vi "4145 validate GUI.vi"(7 "advanced?":bool, 10 "error in (no error)":errorcluster, 11 "AdvancedConfig":T1={"X Axis Name"="", "X axis"=TRUE, "X scale"=TRUE, "Is X axis VAR 1?"=FALSE, "X Axis min"=0.0, "X Axis max"=1.0, "Y1 Axis Name"="", "Y1 scale"=TRUE, "Is VAR 2 used?"=FALSE, "# of steps for VAR 2"=0, "Y1 Axis min"=0.0, "Y1 Axis max"=0.01, "Y2 Axis Name"="", "Y2 axis"=FALSE, "Y2 scale"=TRUE, "Y2 Axis min"=0.0, "Y2 Axis max"=0.01} caption="Simple" {"Y2 Axis max" format="%^.3e"; "Y2 Axis min" format="%^.3e"; "Y1 Axis max" format="%^.3e"; "Y1 Axis min" format="%^.3e"; "X Axis max" format="%^.3e"; "X Axis min" format="%^.3e"}) -> (2 "error out":errorcluster, 3 "valid":bool)   [LabVIEW 2014]
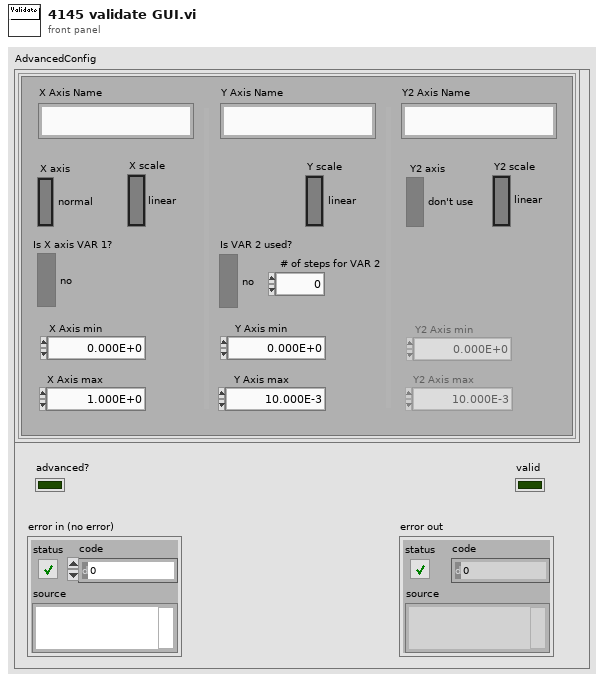
[diagram p1: front panel]
types:
  T1 = cluster{"X Axis Name":string, "X axis":bool, "X scale":bool, "Is X axis VAR 1?":bool, "X Axis min":dbl, "X Axis max":dbl, "Y1 Axis Name":string, "Y1 scale":bool, "Is VAR 2 used?":bool, "# of steps for VAR 2":u16, "Y1 Axis min":dbl, "Y1 Axis max":dbl, "Y2 Axis Name":string, "Y2 axis":bool, "Y2 scale":bool, "Y2 Axis min":dbl, "Y2 Axis max":dbl}
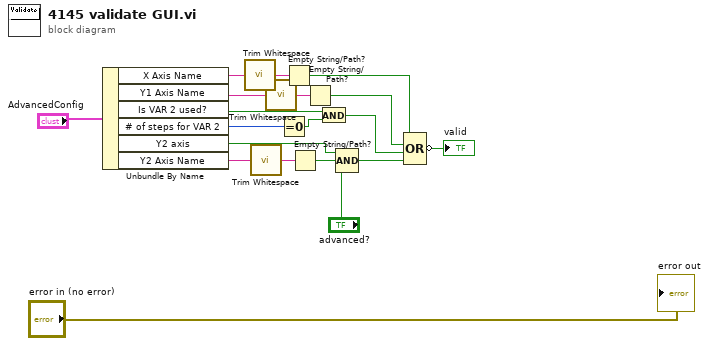
[diagram p0: block diagram]
diagram:
  n1 = Unbundle By Name("AdvancedConfig") -> ("X Axis Name"=w16:string, "Y1 Axis Name"=w12:string, "Is VAR 2 used?"=w6:bool, "# of steps for VAR 2"=w8:u16, "Y2 axis"=w4:bool, "Y2 Axis Name"=w9:string)
  n2 = call <vilib>:"Trim Whitespace.vi"("string"=w16) -> ("trimmed string"=w15:string)  [unwired: 1 in]
  n3 = call <vilib>:"Trim Whitespace.vi"("string"=w9) -> ("trimmed string"=w10:string)  [unwired: 1 in]
  n4 = call <vilib>:"Trim Whitespace.vi"("string"=w12) -> ("trimmed string"=w13:string)  [unwired: 1 in]
  n5 = Equal To 0?(x=w8) -> (x = 0?=w7:bool)
  n6 = Empty String/Path?(string/path=w15) -> (empty?=w14:bool)
  n7 = Empty String/Path?(string/path=w10) -> (empty?=w3:bool)
  n8 = Empty String/Path?(string/path=w13) -> (empty?=w11:bool)
  n9 = And(x=w6, y=w7) -> (x .and. y?=w5:bool)
  n10 = Compound Arithmetic op=AND(w4, w3, "advanced?") -> (w1:bool)
  n11 = Compound Arithmetic op=OR(w14, w11, w5, w1) -> (invert →"valid":bool)
  "error out" <- "error in (no error)"
